vi "MessageBase.setFieldLength.vi"(8 "error in (no error)":errorcluster, 9 "Length":i32, 10 "FIeld.Name":string="Length", 11 "MessageBase in":refnum<class "MessageBase.lvclass">) -> (0 "error out":errorcluster, 3 "MessageBase out":refnum<class "MessageBase.lvclass">)   [LabVIEW 2022 SP3, in "MessageBase.lvclass"]
uses:
  MessageBase.lvclass
  MessageBase.lvclass/MessageBase.ctl
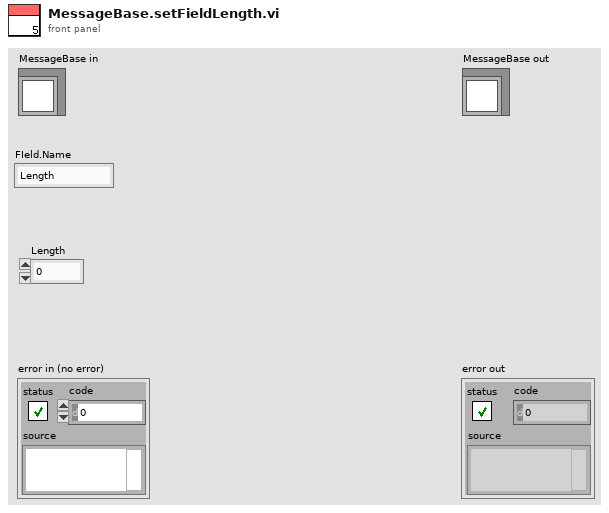
[diagram p1: front panel]
types:
  T1 = typedef "FieldSpec.ctl" = cluster{"Name":string, "Offset":i32, "Length":i32, "FieldType":enum16{"Alphanumeric", "Binary", "BinaryLongPrice", "BinaryShortPrice", "BitField", "PrintableAscii", "Value"}, "FieldValue":variant}
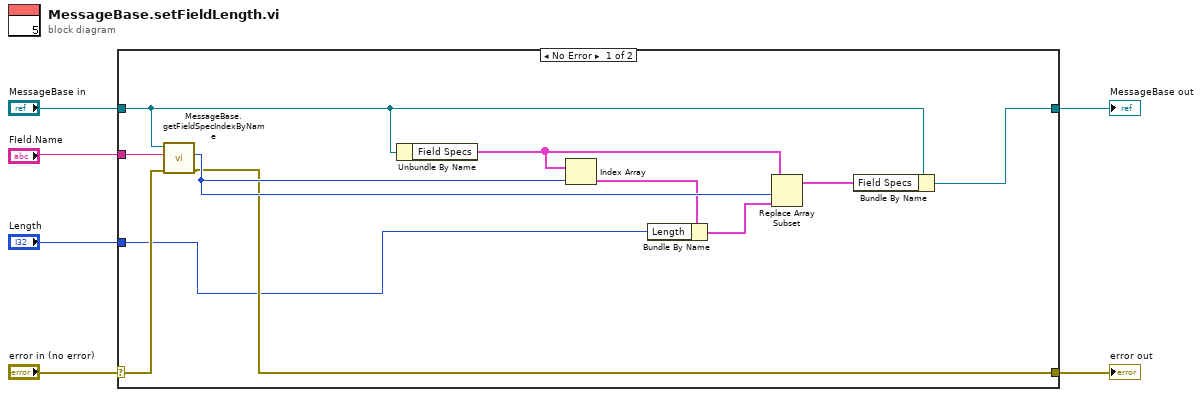
[diagram p0: block diagram]
diagram:
  n1 = case shown="No Error" "error in (no error)" {
    selector: "error in (no error)" -> [w9 w18]
    tunnel: [w8 w18] -> w5
    tunnel: [w10 w19] -> w3
    tunnel: "MessageBase in" -> [w11 w19]
    tunnel: "FIeld.Name" -> [w16 _]
    tunnel: "Length" -> [w7 _]
    frame No Error {
      n2 = call-dynamic "MessageBase.getFieldSpecIndexByName.vi"("error in (no error)"=w9, "Field.Name"=w16, "MessageBase in"=w11) -> ("error out"=w8:errorcluster, "Index"=w14:i32)  [unwired: 6 in, 1 out]
      n3 = Unbundle By Name(w11) -> ("Field Specs"=w15:T1[])
      n4 = Index Array(array=w15, index=w14) -> (element=w13:T1)
      n5 = Bundle By Name(cluster=w13, "Length"=w7) -> (w12:T1)
      n6 = Replace Array Subset(array=w15, new element=w12, index=w14) -> (w17:T1[])
      n7 = Bundle By Name(cluster=w11, "Field Specs"=w17) -> (w10:refnum<class "MessageBase.lvclass">)
    }
    frame Error {
      # "Wire the error cluster across even in the \"No Error\"\ncase so that warnings get propagated."
    }
  }
  "error out" <- w5
  "MessageBase out" <- w3
